vi "newVolume.vi"(10 "scan info":T2, 11 "reader status in":T1) -> (3 "reader status out":T1)   [LabVIEW 2010]
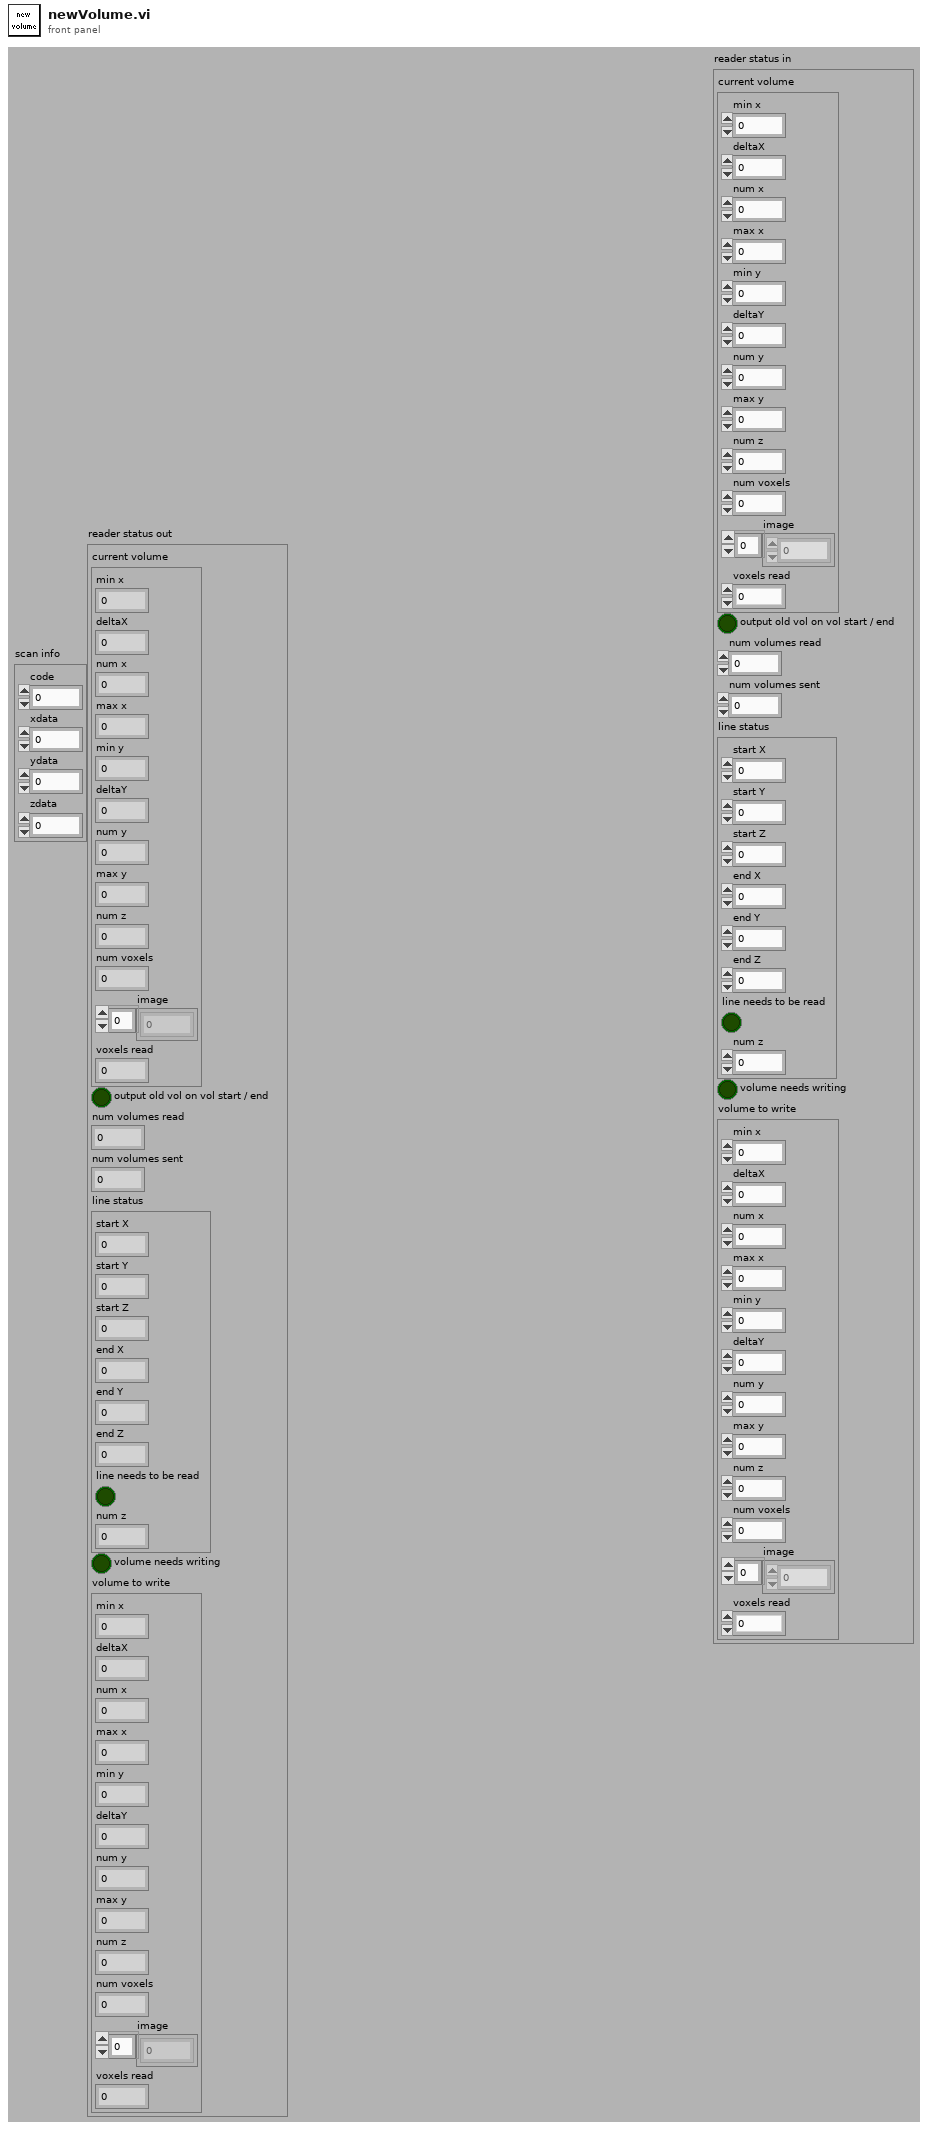
[diagram p1: front panel]
types:
  T1 = cluster{"current volume":cluster{"min x":i16, "deltaX":dbl, "num x":u32, "max x":i16, "min y":i16, "deltaY":dbl, "num y":u32, "max y":i16, "num z":u32, "num voxels":u32, "image":u32[], "voxels read":u32}, "output old vol on vol start / end":bool, "num volumes read":u32, "num volumes sent":u32, "line status":cluster{"start X":i16, "start Y":i16, "start Z":i16, "end X":i16, "end Y":i16, "end Z":i16, "line needs to be read":bool, "num z":u8}, "volume needs writing":bool, "volume to write":cluster{"min x":i16, "deltaX":dbl, "num x":u32, "max x":i16, "min y":i16, "deltaY":dbl, "num y":u32, "max y":i16, "num z":u32, "num voxels":u32, "image":u32[], "voxels read":u32}}
  T2 = cluster{"code":i32, "xdata":i32, "ydata":i32, "zdata":i32}
  T3 = enum16{"NONE", "VOLUME_START", "LINE_START", "LINE_END", "VOLUME_END"}
  T4 = cluster{"min x":i16, "deltaX":dbl, "num x":u32, "max x":i16, "min y":i16, "deltaY":dbl, "num y":u32, "max y":i16, "num z":u32, "num voxels":u32, "image":u32[], "voxels read":u32}
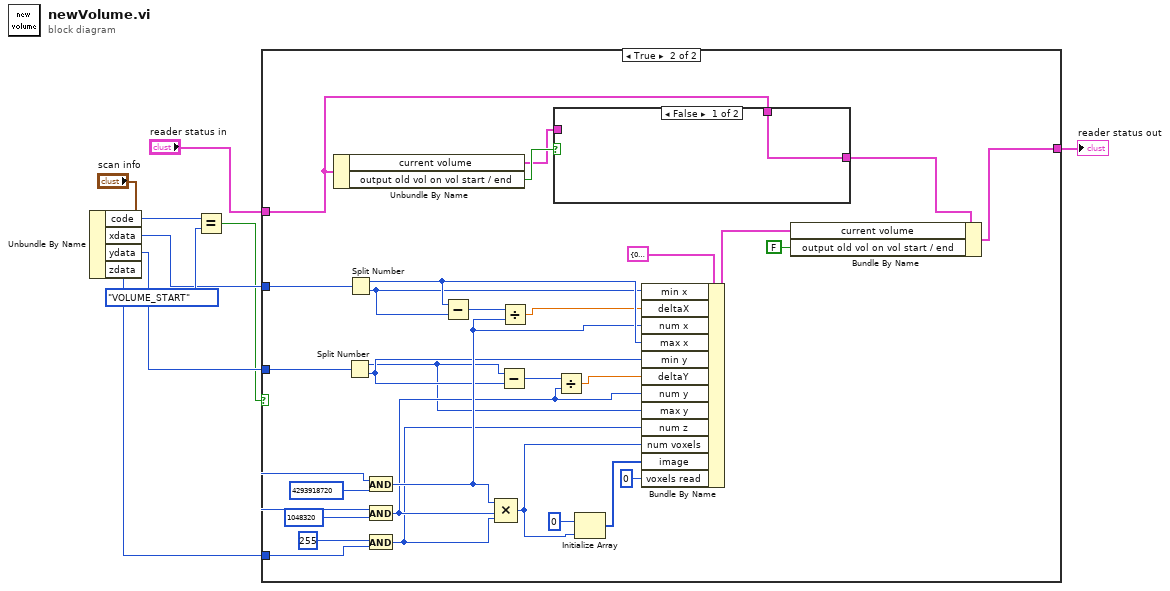
[diagram p0: block diagram]
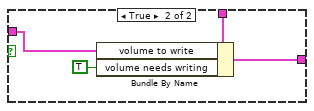
[diagram p3: hidden frame]
diagram:
  n1 = Unbundle By Name("scan info") -> ("code"=w8:i32, "xdata"=w6:i32, "ydata"=w5:i32, "zdata"=w4:i32)
  n2 = Equal?(x=w8, y=T3."VOLUME_START" ("message")) -> (x = y?=w2:bool)
  n3 = case shown="True" w2 {
    tunnel: w6 -> [_ w38]
    tunnel: w5 -> [_ w37]
    tunnel: w4 -> [_ w33]
    tunnel: "reader status in" -> [w10 w13]
    tunnel: [w10 w11] -> w1
    frame False {
    }
    frame True {
      n4 = Unbundle By Name(w13) -> ("current volume"=w14:T4, "output old vol on vol start / end"=w15:bool)
      n5 = Split Number(x=w37) -> (hi(x)=w23:u16, lo(x)=w26:u16)
      n6 = Split Number(x=w38) -> (hi(x)=w30:u16, lo(x)=w28:u16)
      n7 = And(x=w33, y=u32 4293918720) -> (x .and. y?=w29:u32)
      n8 = And(x=w33, y=u32 1048320) -> (x .and. y?=w24:u32)
      n9 = And(x=u32 255, y=w33) -> (x .and. y?=w22:u32)
      n10 = Subtract(x=w30, y=w28) -> (x-y=w32:u16)
      n11 = Compound Arithmetic op=MULTIPLY(w29, w24, w22) -> (w21:u32)
      n12 = Subtract(x=w23, y=w26) -> (x-y=w31:u16)
      n13 = Divide(x=w32, y=w29) -> (x/y=w27:dbl)
      n14 = case shown="False" w15 {
        tunnel: w14 -> [_ w44]
        tunnel: [w40 w42] -> w12
        tunnel: w13 -> [w40 w41]
        frame False {
        }
        frame True {
          n15 = Bundle By Name(cluster=w41, "volume to write"=w44, "volume needs writing"=TRUE) -> (w42:T1)
        }
      }
      n16 = Divide(x=w31, y=w24) -> (x/y=w25:dbl)
      n17 = Initialize Array(u32 0, w21) -> (w19:u32[])
      n18 = Bundle By Name(cluster=T4 {"min x"=0, "deltaX"=0.0, "num x"=0, "max x"=0, "min y"=0, "deltaY"=0.0, "num y"=0, "max y"=0, "num z"=0, "num voxels"=0, "image"=[], "voxels read"=0} ("current volume"), "min x"=w28, "deltaX"=w27, "num x"=w29, "max x"=w30, "min y"=w26, "deltaY"=w25, "num y"=w24, "max y"=w23, "num z"=w22, "num voxels"=w21, "image"=w19, "voxels read"=u32 0) -> (w17:T4)
      n19 = Bundle By Name(cluster=w12, "current volume"=w17, "output old vol on vol start / end"=FALSE) -> (w11:T1)
    }
  }
  "reader status out" <- w1
